vi "Find Subordinate.vi"(7 "Identifier":string, 8 "error in (no error)":errorcluster, 11 "Managed Actor in":refnum<class "Managed Actor.lvclass">) -> (0 "error out":errorcluster, 1 "Queue":refnum<class "Message Enqueuer.lvclass">, 2 "not found?":bool, 3 "Managed Actor out":refnum<class "Managed Actor.lvclass">, 4 "PanelIndex":i32)   [LabVIEW 2023, in "Engine.lvlib" / "Managed Actor.lvlib" / "Managed Actor.lvclass"]
doc: "<b>Find Subordiate</b>\nSearches the map of subordinates for the named actor. If found, it will return the subordinate's data records, and the <b>not found?</b> flag will be false\n\nIf the record is missing,<b>not found?</b> will be true, and the reference data will be invalid"
uses:
  Library/Managed Actor.lvclass
  builds/Framework/Actor Framework.lvlibp/1abvi3w/vi.lib/ActorFramework/Message Enqueuer/Message Enqueuer.lvclass
  Library/Managed Actor.lvclass/Managed Actor.ctl
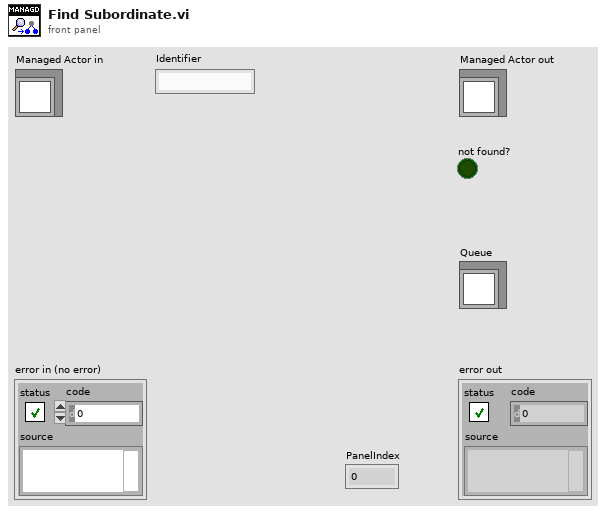
[diagram p1: front panel]
types:
  T1 = typedef "Engine.lvlib/Managed Actor.lvlib/Managed Actor.lvclass/Subordinate.ctl" = cluster{"Identifier":string, "Queue":refnum<class "Message Enqueuer.lvclass">, "PanelIndex":i32}
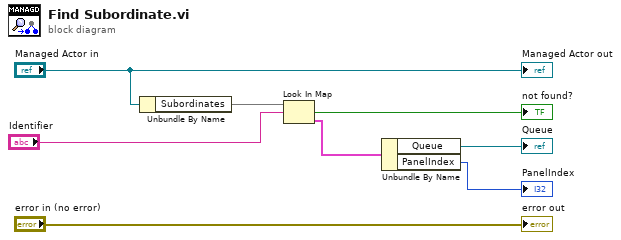
[diagram p0: block diagram]
diagram:
  n1 = Unbundle By Name("Managed Actor in") -> ("Subordinates"=w6:map{string, T1})
  n2 = Look In Map(map=w6, key="Identifier") -> (key not found?=→"not found?":bool, value=w3:T1)  [unwired: 1 in]
  n3 = Unbundle By Name(w3) -> ("Queue"=→"Queue":refnum<class "Message Enqueuer.lvclass">, "PanelIndex"=→"PanelIndex":i32)
  "error out" <- "error in (no error)"
  "Managed Actor out" <- "Managed Actor in"
